vi "Example - Error Meta.vi"() -> ()   [LabVIEW 2016, in "SLL Debug.lvlib"]
uses:
  SLL Debug.lvlib
  <vilib>/Utility/error.llb/Error Cluster From Error Code.vi
  <vilib>/ErrorRing/Error Ring.xnode
panel:
  in  "System Cluster":T1={"Numeric"=123.0, "Boolean"=TRUE, "String"="Hello World!", "System Array"=[0, 1, 2, 3]}
  # "Run this VI to see the SLL Error Meta VI in Action"
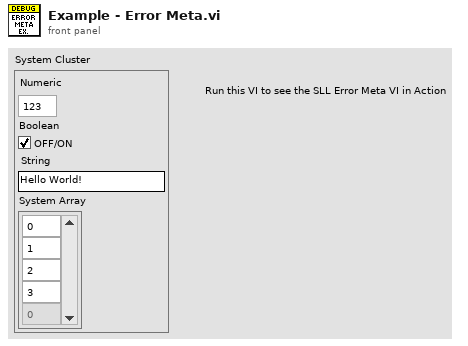
[diagram p1: front panel]
types:
  T1 = cluster{"Numeric":dbl, "Boolean":bool, "String":string, "System Array":u32[]}
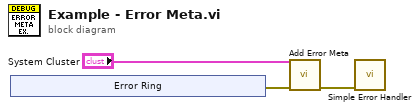
[diagram p0: block diagram]
diagram:
  n1 = xnode "Error Ring"() -> ("error out"=w3:errorcluster)
  n2 = call "Add Error Meta.vi"("error in (no error)"=w3, "Data"="System Cluster") -> ("error out"=w1:errorcluster)  [unwired: 9 in]
  n3 = call <vilib>:"Simple Error Handler.vi"("error in (no error)"=w1) -> ()  [unwired: 4 in, 5 out]
